vi "String to Virtual Key Array.vi"(8 "error in (no error)":errorcluster, 10 "Keyboard Type":u64, 11 "String":string) -> (0 "error out":errorcluster, 3 "Array":u16[](array[numeric]))   [LabVIEW 2020, in "MacroAssert.lvlib" / "Win Util.lvlib"]
uses:
  Win Util.lvlib
  user32.dll
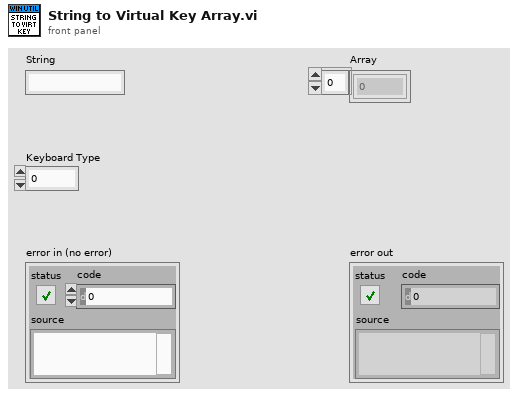
[diagram p1: front panel]
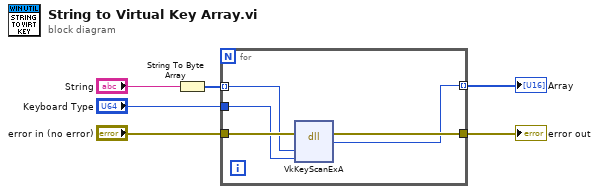
[diagram p0: block diagram]
diagram:
  n1 = String To Byte Array(string="String") -> (unsigned byte array=w3:u8[])
  n2 = for {
    tunnel: [w9] -> w1 mode=indexing
    tunnel: "error in (no error)" -> [w11]
    tunnel: [w10] -> w5
    tunnel: w3 -> [w8] mode=indexing
    tunnel: "Keyboard Type" -> [w7]
    n3 = dll-call lib="user32.dll" fn="VkKeyScanExA"(error in=w11, "TCHAR"=w8, "HKL"=w7) -> (error out=w10:errorcluster, "SHORT"=w9:u16)  [unwired: 4 in, 1 out]
  }
  "error out" <- w5
  "Array" <- w1
